vi "Read Caption.vi"(8 "error in (no error)":errorcluster, 11 "GridColumn in":refnum<class "GridColumn.lvclass">) -> (0 "error out":errorcluster, 2 "Caption":string, 3 "GridColumn out":refnum<class "GridColumn.lvclass">)   [LabVIEW 2016, in "DataGrid.lvlib" / "GridColumn.lvclass"]
uses:
  <userlib>/LabVIEWdotNetDataGrid/source/GridColumn/GridColumn.lvclass
  <userlib>/LabVIEWdotNetDataGrid/source/GridColumn/GridColumn.lvclass/GridColumn.ctl
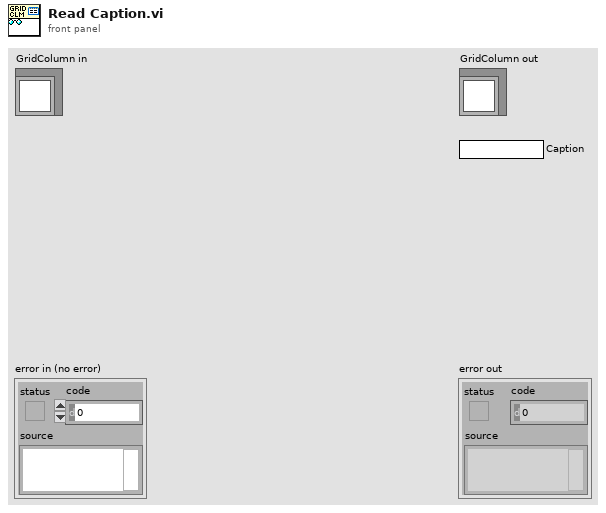
[diagram p1: front panel]
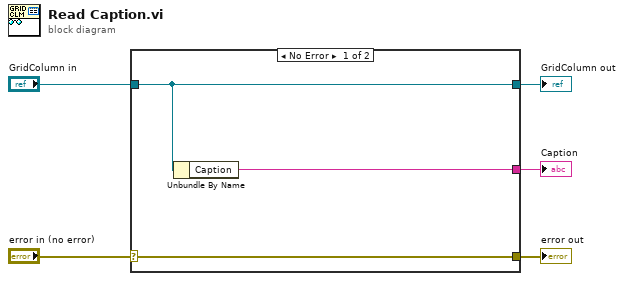
[diagram p0: block diagram]
diagram:
  n1 = case shown="No Error" "error in (no error)" {
    selector: "error in (no error)" -> [w8 w9]
    tunnel: [w8 w9] -> w4
    tunnel: [w7 w10] -> w2
    tunnel: "GridColumn in" -> [w7 w10]
    tunnel: [w6 _] -> w1
    frame No Error {
      n2 = Unbundle By Name(w7) -> ("Caption"=w6:string)
    }
    frame Error {
    }
  }
  "error out" <- w4
  "GridColumn out" <- w2
  "Caption" <- w1
